vi "Keithley 6514 Display Config.vi"(0 "Resource In":refnum<visa-resource-name>, 1 "Check For SCPI Errors? (T)":bool=TRUE, 5 "display  (Display Readings:1)":u16(ring)=1 items=["off", "Display Readings", "Display Text"], 7 "Text To Display":string, 9 "Resolution (digits) (6)":i8=6 min=4 max=7 step=1, 11 "error in (no error)":T1) -> (4 "Resource Out (dupl)":refnum<visa-resource-name>, 15 "error out":T1)   [LabVIEW 2009, in "Keithley 6514 LV 2009.lvlib"]
doc: "This VI is used to configure the display. The VI allows you to put messages up on the display, turn the display off, display normal readings, and control the resolution.\n\ndisplay:\n0 = display enable off\n1 = display readings\n2 = display message test\n\nresolution:\n4 = 4 digits\n5 = 5 digits\n6 = 6 digits\n7 = 7 digits"
uses:
  Keithley 6514 LV 2009.lvlib
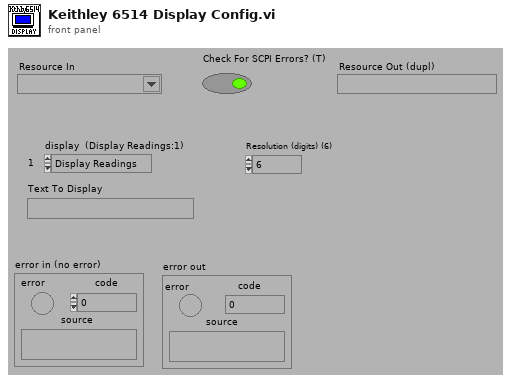
[diagram p1: front panel]
types:
  T1 = cluster{"error":bool, "code":i32, "source":string}
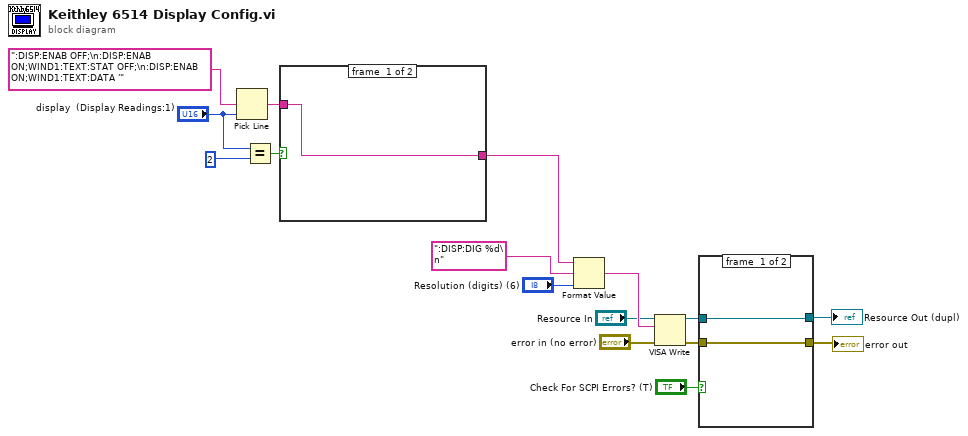
[diagram p0: block diagram]
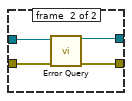
[diagram p2: hidden frame]
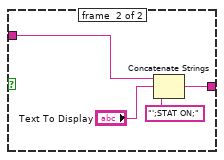
[diagram p3: hidden frame]
diagram:
  n1 = Pick Line(multi-line string=":DISP:ENAB OFF;\n:DISP:ENAB ON;WIND1:TEXT:STAT OFF;\n:DISP:ENAB ON;WIND1:TEXT:DATA '", line index="display  (Display Readings:1)") -> (output string=w9:string)  [unwired: 1 in]
  n2 = Equal?(x="display  (Display Readings:1)", y=u16 2) -> (x = y?=w13:bool)
  n3 = case shown="False" w13 {
    tunnel: [w17 w19] -> w11
    tunnel: w9 -> [w17 w18]
    frame #0 {
    }
    frame #1 {
      n4 = Concatenate Strings(w18, "Text To Display", "';STAT ON;") -> (w19:string)
    }
  }
  n5 = Format Value(string ("")=w11, format string=":DISP:DIG %d\n", value (0)="Resolution (digits) (6)") -> (output string=w7:string)
  n6 = VISA Write(VISA resource name="Resource In", write buffer=w7, error in (no error)="error in (no error)") -> (VISA resource name out=w4:refnum<visa-resource-name>, error out=w3:errorcluster)  [unwired: 1 out]
  n7 = case shown="False" "Check For SCPI Errors? (T)" {
    tunnel: w4 -> [w23 w27]
    tunnel: w3 -> [w22 w26]
    tunnel: [w23 w25] -> w1
    tunnel: [w22 w24] -> w2
    frame #0 {
    }
    frame #1 {
      n8 = call "Error Query.vi"("VISA Resource In"=w27, "error in (no error)"=w26) -> ("VISA Resource Out (dupl)"=w25:refnum<visa-resource-name>, "error out"=w24:errorcluster)  [unwired: 10 in, 2 out]
    }
  }
  "error out" <- w2
  "Resource Out (dupl)" <- w1
